vi "prepAO_img_old.vi"   [LabVIEW 2015]
uses:
  <vilib>/DAQmx/write.llb/DAQmx Write (Analog 2D DBL NChan NSamp).vi
  <vilib>/DAQmx/create/channels.llb/DAQmx Create Channel (AO-Voltage-Basic).vi
  <vilib>/DAQmx/configure/timing.llb/DAQmx Timing (Sample Clock).vi
  <vilib>/DAQmx/miscellaneous.llb/DAQmx Fill In Error Info.vi
types:
  T1 = typedef "LVRectTypeDef.ctl" = cluster{"Left":i16, "Top":i16, "Right":i16, "Bottom":i16}
  T2 = cluster{"Xpixels":i32, "Vxminref":dbl, "Vxmaxref":dbl, "P":dbl, "Ypixels":i32, "Vyminref":dbl, "Vymaxref":dbl, "srate":sgl, "sAOxy":i32, "timeout":dbl, "type":string, "date":string, "time":string, "Colormap":u16, "Drawing Mode":u16, "Scanning Mode":u16, "square pixels":bool, "square matrix":bool, "Xpixels Img":i32, "Vx-min Img":dbl, "VX-max Img":dbl, "Ypixels Img":i32, "Vy-min Img":dbl, "Vy-max Img ":dbl, "Angle Img":dbl, "autoshutter":bool, "finite":bool, "cont":bool, "wavdet":bool, "measpoints":i32, "avpp":i32, "bufferAO":i32, "bufferAI":i32, "CH1":bool, "CH2":bool, "X":bool, "Y":bool, "Ip":bool, "Vp":bool, "starttick":u32, "waveform":path, "Vx-ref":dbl, "Vy-ref":dbl, "refreshrate":dbl, "refreshbuffer":i32, "tt_cycles":i32, "motorref":refnum<k7>, "mirrorswitch":refnum<k7>, "sample mode":i32, "maxbufferAI":i32, "sampletreshold":dbl, "srateAODO":sgl, "bin":sgl, "Pel":sgl, "Angle draw":dbl, "srate Img":sgl, "ROIimg_plotbounds":T1, "auto OD":bool, "ODfilt":u16, "reset AO_DO":bool}
  T3 = cluster{"CH1 AI":tag, "CH1 CI":tag, "CH2 AI":tag, "CH2 CI":tag, "AI X":tag, "AI Y":tag, "AO X-Y":tag, "CH1ST":bool, "CH2ST":bool, "Sigcase":i16, "StageS":i32, "StageL":i32, "data dir":path, "Vp":tag, "Ip":tag, "AO CWlaser":tag, "AO VtoP":tag, "shutter":tag, "488":tag, "532":tag, "640":tag, "LT marker":tag, "image OD":u16, "contour OD":u16, "point OD":u16}
  T4 = cluster{"Min Voltage sq (mV)":dbl, "Max voltage sq (mV)":dbl, "Duty cycle sq(%)":dbl, "Voltage freq. sq(Hz)":dbl, "# cycles sq":u32, "meastype":enum16{"sealtest hekcells", "sealtest neurons", "Manual", "from file"}, "sample rate":dbl, "amp":dbl, "sample mode":i32, "refreshbuffer":i32, "timeout":sgl, "patch":bool, "laserAO":bool, "shutter":bool, "488":bool, "532":bool, "640":bool, "LT marker":bool, "Min Voltage tri (mV)":dbl, "Max voltage tri (mV)":dbl, "Voltage freq. tri(Hz)":dbl, "# cycles tri":u32, "Voltage step ":bool, "Voltage triangle":bool, "file":bool, "refreshrate":dbl, "sAOXY":dbl, "avpp":i32, "Pel":dbl, "bin":dbl}
  T5 = cluster{"VtoP":sgl[], "CWlasers":sgl[], "shutter":sgl[], "488":sgl[], "532":sgl[], "640":sgl[], "LT marker":sgl[]}
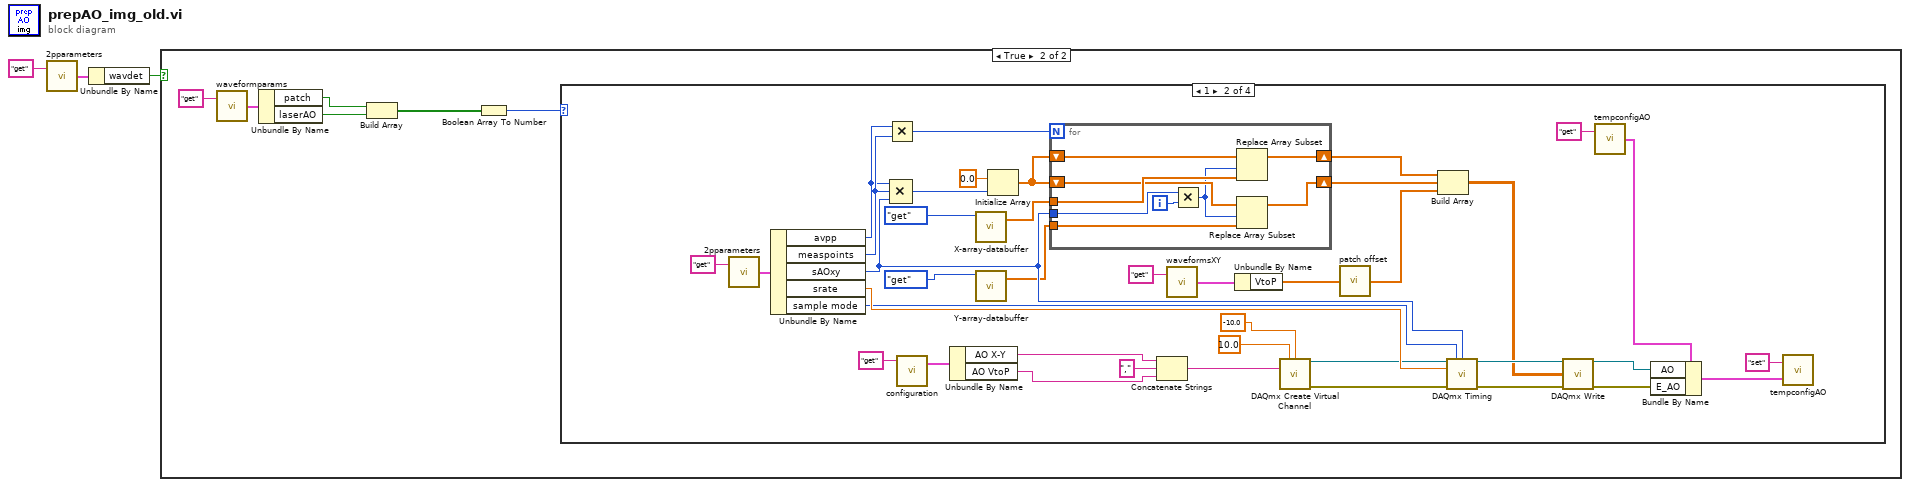
[diagram p0: block diagram]
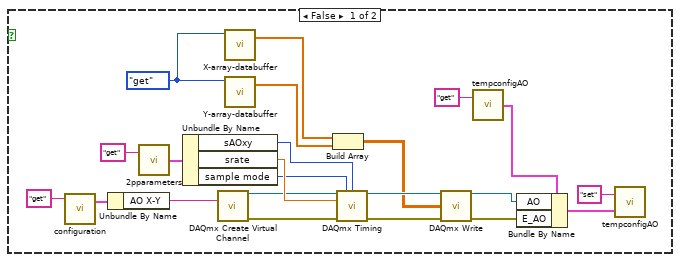
[diagram p2: hidden frame]
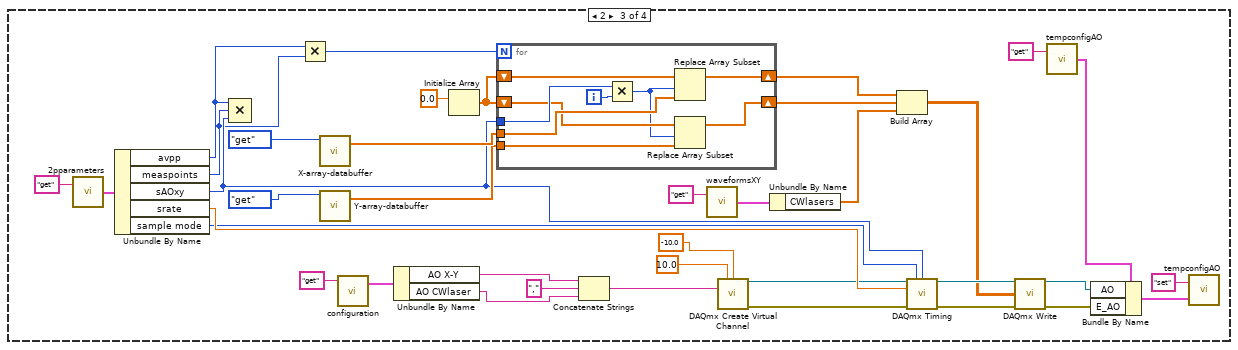
[diagram p4: hidden frame]
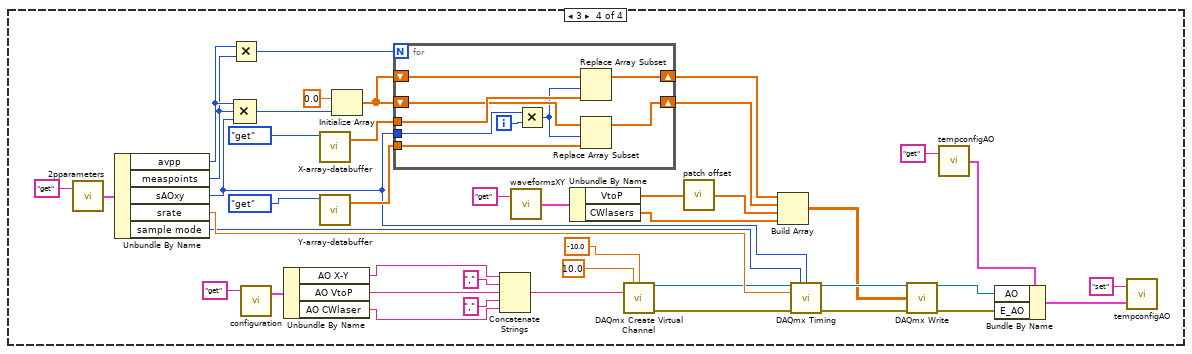
[diagram p5: hidden frame]
diagram:
  n1 = call "2pparameters.vi"("command"="get") -> ("Params out"=w2:T2)  [unwired: 1 in]
  n2 = Unbundle By Name(w2) -> ("wavdet"=w1:bool)
  n3 = case shown="True" w1 {
    frame False {
      w18 = enum16{"get", "set", "clear", "append"}."get" ("command")
      n4 = call "configuration.vi"("command"="get") -> ("config out"=w19:T3)  [unwired: 2 in, 1 out]
      n5 = Unbundle By Name(w19) -> ("AO X-Y"=w21:tag)
      n6 = call "2pparameters.vi"("command"="get") -> ("Params out"=w23:T2)  [unwired: 1 in]
      n7 = Unbundle By Name(w23) -> ("sAOxy"=w24:i32, "srate"=w25:sgl, "sample mode"=w15:i32)
      n8 = call-poly <vilib>:"DAQmx Create Virtual Channel.vi"("physical channels"=w21) -> ("task out"=w7:refnum<k21>, "error out"=w6:errorcluster)  [unwired: 13 in]
      n9 = call "X-array-databuffer.vi"("command"=w18) -> ("array out"=w5:dbl[])  [unwired: 3 in, 1 out]
      n10 = call "Y-array-databuffer.vi"("command"=w18) -> ("array out"=w4:dbl[])  [unwired: 3 in, 1 out]
      n11 = Build Array(w5, w4) -> (w14:dbl[][])
      n12 = call-poly <vilib>:"DAQmx Timing.vi"("task/channels in"=w7, "sample mode"=w15, "samples per channel"=w24, "rate"=w25, "error in"=w6) -> ("task out"=w17:refnum<k21>, "error out"=w16:errorcluster)  [unwired: 9 in]
      n13 = call-poly <vilib>:"DAQmx Write.vi"("task/channels in"=w17, "data"=w14, "error in"=w16) -> ("task out"=w9:refnum<k21>, "error out"=w8:errorcluster)  [unwired: 10 in, 1 out]
      n14 = call "tempconfigAO.vi"("command"="get") -> ("Temp Config out"=w12:cluster{"AO":refnum<k21>, "E_AO":errorcluster})  [unwired: 1 in]
      n15 = Bundle By Name(cluster=w12, "AO"=w9, "E_AO"=w8) -> (w13:cluster{"AO":refnum<k21>, "E_AO":errorcluster})
      n16 = call "tempconfigAO.vi"("Temp Config in"=w13, "command"="set") -> ()  [unwired: 1 out]
    }
    frame True {
      n17 = call "waveformparams.vi"("command"="get") -> ("Params out"=w29:T4)  [unwired: 1 in]
      n18 = Unbundle By Name(w29) -> ("patch"=w28:bool, "laserAO"=w27:bool)
      n19 = Build Array(w28, w27) -> (w26:bool[])
      n20 = Boolean Array To Number(Boolean array=w26) -> (number=w31:u32)
      n21 = case shown="1" w31 {
        frame 0, Default {
        }
        frame 1 {
          n22 = call "2pparameters.vi"("command"="get") -> ("Params out"=w65:T2)  [unwired: 1 in]
          n23 = Unbundle By Name(w65) -> ("avpp"=w32:i32, "measpoints"=w34:i32, "sAOxy"=w44:i32, "srate"=w66:sgl, "sample mode"=w58:i32)
          n24 = Multiply(x=w32, y=w34) -> (x*y=w33:i32)
          n25 = Compound Arithmetic op=MULTIPLY(w32, w34, w44) -> (w45:i32)
          n26 = call "configuration.vi"("command"="get") -> ("config out"=w62:T3)  [unwired: 2 in, 1 out]
          n27 = Unbundle By Name(w62) -> ("AO X-Y"=w54:tag, "AO VtoP"=w53:tag)
          n28 = call "X-array-databuffer.vi"("command"=enum16{"get", "set", "clear", "append"}."get") -> ("array out"=w43:dbl[])  [unwired: 3 in, 1 out]
          n29 = call "Y-array-databuffer.vi"("command"=enum16{"get", "set", "clear", "append"}."get") -> ("array out"=w41:dbl[])  [unwired: 3 in, 1 out]
          n30 = Initialize Array(0.0 ("element"), w45) -> (w42:dbl[])
          n31 = for {
            N: w33 -> [_]
            shift-right: [w77] -> w40
            shift-left: w42 -> [w80]
            tunnel: w44 -> [w79]
            tunnel: w43 -> [w76]
            shift-right: [w74] -> w39
            shift-left: w42 -> [w75]
            tunnel: w41 -> [w72]
            i -> [w78]
            n32 = Multiply(x=w79, y=w78) -> (x*y=w73:i32)
            n33 = Replace Array Subset(array=w80, new element=w76, index=w73) -> (w77:dbl[])
            n34 = Replace Array Subset(array=w75, new element=w72, index=w73) -> (w74:dbl[])
          }
          n35 = Concatenate Strings(w54, "," ("string"), w53) -> (w52:string)
          n36 = call "waveformsXY.vi"("command"="get") -> ("waveforms out"=w35:T5)  [unwired: 1 in]
          n37 = Unbundle By Name(w35) -> ("VtoP"=w37:sgl[])
          n38 = call-poly <vilib>:"DAQmx Create Virtual Channel.vi"("maximum value"=10.0, "minimum value"=-10.0, "physical channels"=w52) -> ("task out"=w48:refnum<k21>, "error out"=w47:errorcluster)  [unwired: 11 in]
          n39 = call "patch offset.vi"("VtoPin"=w37) -> ("VtoPout"=w36:dbl[])
          n40 = Build Array(w40, w39, w36) -> (w51:dbl[][])
          n41 = call-poly <vilib>:"DAQmx Timing.vi"("task/channels in"=w48, "sample mode"=w58, "samples per channel"=w44, "rate"=w66, "error in"=w47) -> ("task out"=w60:refnum<k21>, "error out"=w59:errorcluster)  [unwired: 9 in]
          n42 = call-poly <vilib>:"DAQmx Write.vi"("task/channels in"=w60, "data"=w51, "error in"=w59) -> ("task out"=w49:refnum<k21>, "error out"=w50:errorcluster)  [unwired: 10 in, 1 out]
          n43 = call "tempconfigAO.vi"("command"="get") -> ("Temp Config out"=w70:cluster{"AO":refnum<k21>, "E_AO":errorcluster})  [unwired: 1 in]
          n44 = Bundle By Name(cluster=w70, "AO"=w49, "E_AO"=w50) -> (w71:cluster{"AO":refnum<k21>, "E_AO":errorcluster})
          n45 = call "tempconfigAO.vi"("Temp Config in"=w71, "command"="set") -> ()  [unwired: 1 out]
        }
        frame 2 {
          n46 = call "2pparameters.vi"("command"="get") -> ("Params out"=w111:T2)  [unwired: 1 in]
          n47 = Unbundle By Name(w111) -> ("avpp"=w82:i32, "measpoints"=w81:i32, "sAOxy"=w83:i32, "srate"=w112:sgl, "sample mode"=w105:i32)
          n48 = Compound Arithmetic op=MULTIPLY(w82, w81, w83) -> ()  [unwired: 1 out]
          n49 = Multiply(x=w82, y=w81) -> (x*y=w84:i32)
          n50 = call "X-array-databuffer.vi"("command"=enum16{"get", "set", "clear", "append"}."get") -> ("array out"=w90:dbl[])  [unwired: 3 in, 1 out]
          n51 = call "Y-array-databuffer.vi"("command"=enum16{"get", "set", "clear", "append"}."get") -> ("array out"=w88:dbl[])  [unwired: 3 in, 1 out]
          n52 = call "configuration.vi"("command"="get") -> ("config out"=w108:T3)  [unwired: 2 in, 1 out]
          n53 = Unbundle By Name(w108) -> ("AO X-Y"=w102:tag, "AO CWlaser"=w95:tag)
          n54 = Initialize Array(0.0 ("element")) -> (w89:dbl[])  [unwired: 1 in]
          n55 = for {
            N: w84 -> [_]
            shift-right: [w124] -> w86
            shift-left: w89 -> [w127]
            tunnel: w83 -> [w126]
            tunnel: w90 -> [w123]
            shift-right: [w121] -> w85
            shift-left: w89 -> [w122]
            tunnel: w88 -> [w119]
            i -> [w125]
            n56 = Multiply(x=w126, y=w125) -> (x*y=w120:i32)
            n57 = Replace Array Subset(array=w127, new element=w123, index=w120) -> (w124:dbl[])
            n58 = Replace Array Subset(array=w122, new element=w119, index=w120) -> (w121:dbl[])
          }
          n59 = Concatenate Strings(w102, "," ("string"), w95) -> (w101:string)
          n60 = call "waveformsXY.vi"("command"="get") -> ("waveforms out"=w118:T5)  [unwired: 1 in]
          n61 = call-poly <vilib>:"DAQmx Create Virtual Channel.vi"("maximum value"=10.0, "minimum value"=-10.0, "physical channels"=w101) -> ("task out"=w94:refnum<k21>, "error out"=w93:errorcluster)  [unwired: 11 in]
          n62 = Unbundle By Name(w118) -> ("CWlasers"=w97:sgl[])
          n63 = Build Array(w86, w85, w97) -> (w100:dbl[][])
          n64 = call-poly <vilib>:"DAQmx Timing.vi"("task/channels in"=w94, "sample mode"=w105, "samples per channel"=w83, "rate"=w112, "error in"=w93) -> ("task out"=w107:refnum<k21>, "error out"=w106:errorcluster)  [unwired: 9 in]
          n65 = call-poly <vilib>:"DAQmx Write.vi"("task/channels in"=w107, "data"=w100, "error in"=w106) -> ("task out"=w98:refnum<k21>, "error out"=w99:errorcluster)  [unwired: 10 in, 1 out]
          n66 = call "tempconfigAO.vi"("command"="get") -> ("Temp Config out"=w115:cluster{"AO":refnum<k21>, "E_AO":errorcluster})  [unwired: 1 in]
          n67 = Bundle By Name(cluster=w115, "AO"=w98, "E_AO"=w99) -> (w116:cluster{"AO":refnum<k21>, "E_AO":errorcluster})
          n68 = call "tempconfigAO.vi"("Temp Config in"=w116, "command"="set") -> ()  [unwired: 1 out]
        }
        frame 3 {
          n69 = call "2pparameters.vi"("command"="get") -> ("Params out"=w163:T2)  [unwired: 1 in]
          n70 = Unbundle By Name(w163) -> ("avpp"=w130:i32, "measpoints"=w129:i32, "sAOxy"=w132:i32, "srate"=w164:sgl, "sample mode"=w157:i32)
          n71 = Multiply(x=w130, y=w129) -> (x*y=w131:i32)
          n72 = Compound Arithmetic op=MULTIPLY(w130, w129, w132) -> (w128:i32)
          n73 = call "configuration.vi"("command"="get") -> ("config out"=w160:T3)  [unwired: 2 in, 1 out]
          n74 = Unbundle By Name(w160) -> ("AO X-Y"=w153:tag, "AO VtoP"=w152:tag, "AO CWlaser"=w145:tag)
          n75 = call "X-array-databuffer.vi"("command"=enum16{"get", "set", "clear", "append"}."get") -> ("array out"=w140:dbl[])  [unwired: 3 in, 1 out]
          n76 = call "Y-array-databuffer.vi"("command"=enum16{"get", "set", "clear", "append"}."get") -> ("array out"=w138:dbl[])  [unwired: 3 in, 1 out]
          n77 = Initialize Array(0.0 ("element"), w128) -> (w139:dbl[])
          n78 = for {
            N: w131 -> [_]
            shift-right: [w176] -> w136
            shift-left: w139 -> [w179]
            tunnel: w132 -> [w178]
            tunnel: w140 -> [w175]
            shift-right: [w173] -> w135
            shift-left: w139 -> [w174]
            tunnel: w138 -> [w171]
            i -> [w177]
            n79 = Multiply(x=w178, y=w177) -> (x*y=w172:i32)
            n80 = Replace Array Subset(array=w179, new element=w175, index=w172) -> (w176:dbl[])
            n81 = Replace Array Subset(array=w174, new element=w171, index=w172) -> (w173:dbl[])
          }
          n82 = Concatenate Strings(w153, "," ("string"), w152, "," ("string"), w145) -> (w151:string)
          n83 = call "waveformsXY.vi"("command"="get") -> ("waveforms out"=w170:T5)  [unwired: 1 in]
          n84 = Unbundle By Name(w170) -> ("VtoP"=w134:sgl[], "CWlasers"=w147:sgl[])
          n85 = call-poly <vilib>:"DAQmx Create Virtual Channel.vi"("maximum value"=10.0, "minimum value"=-10.0, "physical channels"=w151) -> ("task out"=w144:refnum<k21>, "error out"=w143:errorcluster)  [unwired: 11 in]
          n86 = call "patch offset.vi"("VtoPin"=w134) -> ("VtoPout"=w133:dbl[])
          n87 = Build Array(w136, w135, w133, w147) -> (w150:dbl[][])
          n88 = call-poly <vilib>:"DAQmx Timing.vi"("task/channels in"=w144, "sample mode"=w157, "samples per channel"=w132, "rate"=w164, "error in"=w143) -> ("task out"=w159:refnum<k21>, "error out"=w158:errorcluster)  [unwired: 9 in]
          n89 = call-poly <vilib>:"DAQmx Write.vi"("task/channels in"=w159, "data"=w150, "error in"=w158) -> ("task out"=w148:refnum<k21>, "error out"=w149:errorcluster)  [unwired: 10 in, 1 out]
          n90 = call "tempconfigAO.vi"("command"="get") -> ("Temp Config out"=w167:cluster{"AO":refnum<k21>, "E_AO":errorcluster})  [unwired: 1 in]
          n91 = Bundle By Name(cluster=w167, "AO"=w148, "E_AO"=w149) -> (w168:cluster{"AO":refnum<k21>, "E_AO":errorcluster})
          n92 = call "tempconfigAO.vi"("Temp Config in"=w168, "command"="set") -> ()  [unwired: 1 out]
        }
      }
    }
  }
